vi "SphereXYtoZ.vi"(9 "distance from center y":dbl, 10 "Distance from center x":dbl, 11 "Radius":dbl) -> (3 "distance from center Z":dbl)   [LabVIEW 2023]
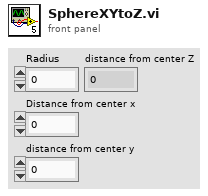
[diagram p1: front panel]
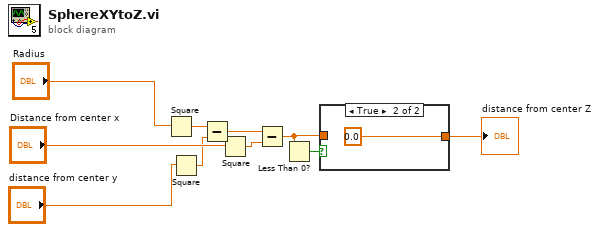
[diagram p0: block diagram]
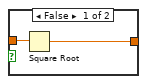
[diagram p2: hidden frame]
diagram:
  n1 = Square(x="Radius") -> (x^2=w4:dbl)
  n2 = Square(x="distance from center y") -> (x^2=w6:dbl)
  n3 = Subtract(x=w4, y=w6) -> (x-y=w7:dbl)
  n4 = Square(x="Distance from center x") -> (x^2=w8:dbl)
  n5 = Subtract(x=w7, y=w8) -> (x-y=w1:dbl)
  n6 = Less Than 0?(x=w1) -> (x < 0?=w2:bool)
  n7 = case shown="True" w2 {
    tunnel: [w12 0.0] -> w10
    tunnel: w1 -> [w11 _]
    frame False {
      n8 = Square Root(x=w11) -> (sqrt(x)=w12:dbl)
    }
    frame True {
    }
  }
  "distance from center Z" <- w10
